vi "swerveTasks.vi"(1 "limitSwitch[]":bool[](array[boolean]), 2 "realGyro":dbl, 3 "steeringEncoderRAW[]":dbl[](array[numeric]), 5 "driveEncoderRAW[]":dbl[](array[numeric]), 6 "driveEncoderSpeeds[]":dbl[](array[numeric])) -> (0 "zeroEncoders":bool[](array[boolean]))   [LabVIEW 2019]
uses:
  swerveData.vi
panel:
  in  "offsets[]":dbl[](array[numeric])=[177.0, 265.0, 355.0, 78.0]
  in  "gyro offset":dbl format="%#_13g"
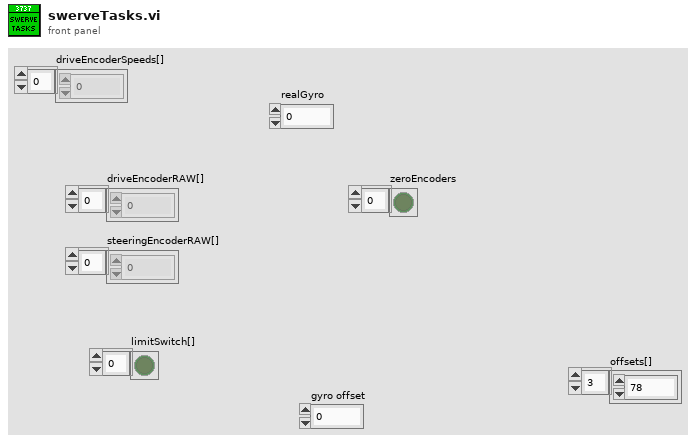
[diagram p1: front panel]
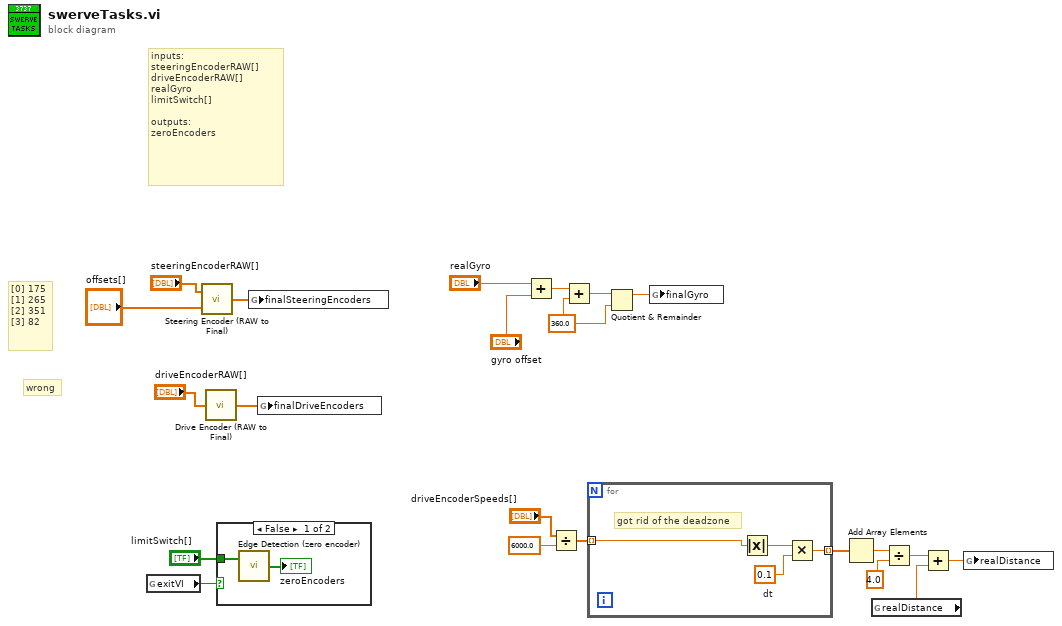
[diagram p0: block diagram]
diagram:
  w14 = 360.0 ("y")
  # "wrong"
  # "[0] 175\n[1] 265\n[2] 351\n[3] 82"
  # "inputs:\nsteeringEncoderRAW[]\ndriveEncoderRAW[]\nrealGyro\nlimitSwitch[]\n\noutputs:\nzeroEncoders"
  n1 = global read "swerveData.vi" "exitVI"() -> (w11:bool)
  n2 = call "Steering Encoder (RAW to Final).vi"("offsets[]"="offsets[]", "encoderRAW[]"="steeringEncoderRAW[]") -> ("finalAngle"=w21:dbl[])
  n3 = call "Drive Encoder (RAW to Final).vi"("encoderRAW[]"="driveEncoderRAW[]") -> ("finalEncoder[]"=w19:dbl[])
  n4 = case shown="False" w11 {
    tunnel: "limitSwitch[]" -> [w24 _]
    frame False {
      n5 = call "Edge Detection (zero encoder).vi"("limitSwitch[]"=w24) -> ("zeroEncoders"=→"zeroEncoders":bool[])  [unwired: 1 in]
    }
    frame True {
    }
  }
  n6 = global write "swerveData.vi" "finalSteeringEncoders"(w21) -> ()
  n7 = global write "swerveData.vi" "finalDriveEncoders"(w19) -> ()
  n8 = Add(x="realGyro", y="gyro offset") -> (x+y=w15:dbl)
  n9 = Divide(x="driveEncoderSpeeds[]", y=6000.0) -> (x/y=w4:dbl[])
  n10 = Add(x=w15, y=w14) -> (x+y=w13:dbl)
  n11 = for {
    tunnel: w4 -> [w25] mode=indexing
    tunnel: [w26] -> w9 mode=indexing
    w27 = 0.1  # dt
    # "got rid of the deadzone"
    n12 = Absolute Value(x=w25) -> (abs(x)=w28:dbl)
    n13 = Multiply(x=w28, y=w27) -> (x*y=w26:dbl)
  }
  n14 = Quotient & Remainder(x=w13, y=w14) -> (x-y*floor(x/y)=w12:dbl)  [unwired: 1 out]
  n15 = global write "swerveData.vi" "finalGyro"(w12) -> ()
  n16 = Add Array Elements(numeric array=w9) -> (sum=w8:dbl)
  n17 = global read "swerveData.vi" "realDistance"() -> (w1:dbl)
  n18 = Divide(x=w8, y=4.0) -> (x/y=w3:dbl)
  n19 = Add(x=w3, y=w1) -> (x+y=w2:dbl)
  n20 = global write "swerveData.vi" "realDistance"(w2) -> ()
